vi "Initialise Ship.vi"(6 "Ship":T1, 8 "error in (no error)":errorcluster, 11 "Renderer":u32) -> (0 "error out":errorcluster, 3 "Ship":refnum<class "Ship.lvclass">)   [LabVIEW 2021, in "Main Controller Actor.lvclass"]
uses:
  Main Controller Actor.lvclass
  Main Controller Actor.lvclass/Main Controller Actor.ctl
  Ships/Arilou/Arilou.lvclass
  C:/dev/LabVIEW/LabMelee/Source/Application Specific/Ship/Ship.lvclass
  C:/dev/LabVIEW/LabMelee/Source/Application Specific/Element/Element.lvclass
  C:/dev/LabVIEW/LabMelee/Source/Application Specific/Ships/Arilou/Arilou.lvclass
  Ships/Chmmr/Chmmr.lvclass
  C:/dev/LabVIEW/LabMelee/Source/Application Specific/Ships/Chmmr/Chmmr.lvclass
  Ships/Kohrah/Kohrah.lvclass
  C:/dev/LabVIEW/LabMelee/Source/Application Specific/Ships/Kohrah/Kohrah.lvclass
  Ships/Slylandro/Slylandro.lvclass
  C:/dev/LabVIEW/LabMelee/Source/Application Specific/Ships/Slylandro/Slylandro.lvclass
  Ship/Ship.lvclass
  Ship.ctl
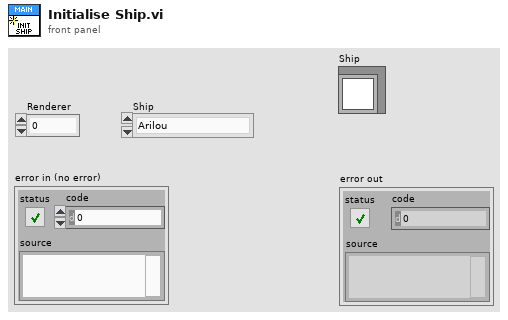
[diagram p1: front panel]
types:
  T1 = typedef "Main Controller Actor.lvclass/Ship.ctl" = enum16{"Arilou", "Chmmr", "Kohrah", "Slylandro"}
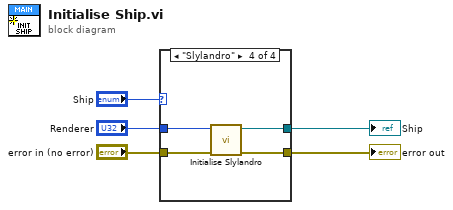
[diagram p0: block diagram]
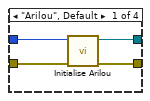
[diagram p2: hidden frame]
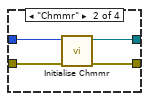
[diagram p3: hidden frame]
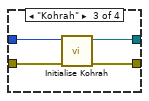
[diagram p4: hidden frame]
diagram:
  n1 = case shown="\"Slylandro\"" "Ship" {
    tunnel: "error in (no error)" -> [w9 w13 w15 w21]
    tunnel: [w8 w12 w16 w20] -> w2
    tunnel: [w7 w11 w17 w19] -> w3
    tunnel: "Renderer" -> [w6 w10 w14 w18]
    frame "Arilou", Default {
      n2 = call "Initialise Arilou.vi"("error in (no error)"=w9, "Renderer"=w6) -> ("error out"=w8:errorcluster, "Ship out"=w7:refnum<class "Arilou.lvclass">)  [unwired: 8 in]
    }
    frame "Chmmr" {
      n3 = call "Initialise Chmmr.vi"("error in (no error)"=w13, "Renderer"=w10) -> ("error out"=w12:errorcluster, "Ship out"=w11:refnum<class "Chmmr.lvclass">)  [unwired: 8 in]
    }
    frame "Kohrah" {
      n4 = call "Initialise Kohrah.vi"("error in (no error)"=w15, "Renderer"=w14) -> ("error out"=w16:errorcluster, "Ship out"=w17:refnum<class "Kohrah.lvclass">)  [unwired: 8 in]
    }
    frame "Slylandro" {
      n5 = call "Initialise Slylandro.vi"("error in (no error)"=w21, "Renderer"=w18) -> ("error out"=w20:errorcluster, "Ship out"=w19:refnum<class "Slylandro.lvclass">)  [unwired: 8 in]
    }
  }
  "error out" <- w2
  "Ship" <- w3
